vi "Handle Error.vi"(8 "error in (no error)":errorcluster, 11 "Module Data In":refnum<class "Rename.lvclass">) -> (0 "error out":errorcluster, 2 "Stop Module":bool, 3 "Module Data Out":refnum<class "Rename.lvclass">)   [LabVIEW 2015, in "Generic Module Library.lvlib" / "Template G_Module.lvlib" / "Rename.lvclass"]
uses:
  Rename.lvclass
  Template G_Module.lvlib
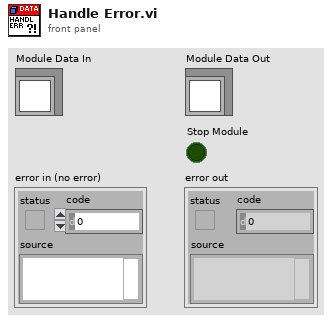
[diagram p1: front panel]
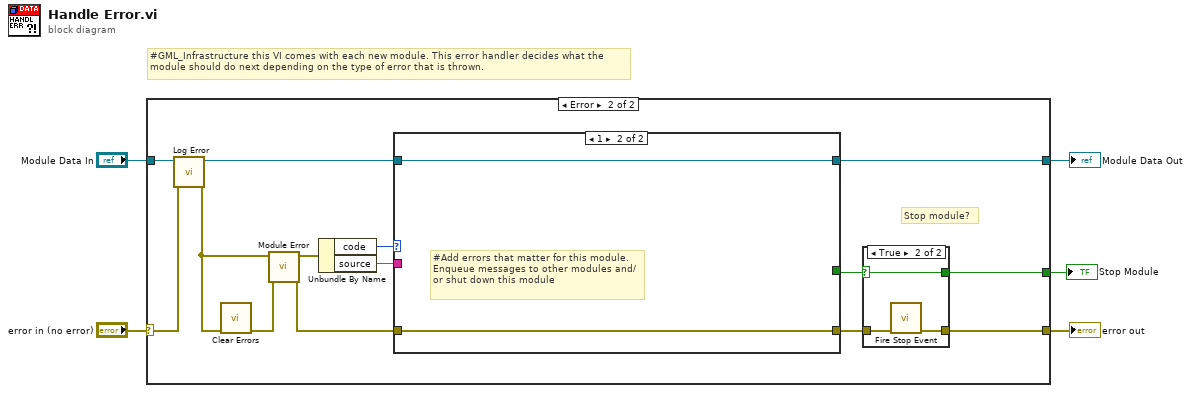
[diagram p0: block diagram]
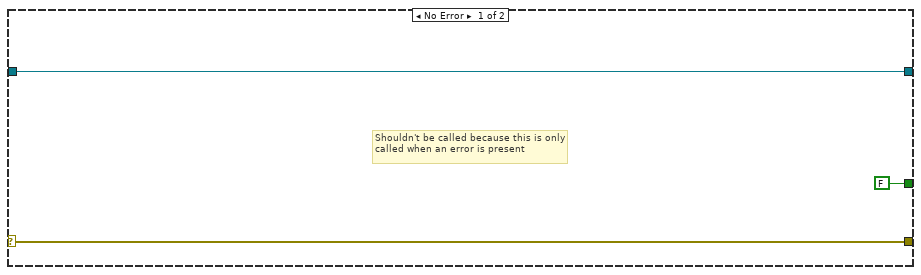
[diagram p2: hidden frame]
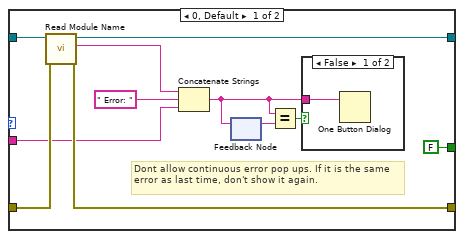
[diagram p4: hidden frame]
diagram:
  # "#GML_Infrastructure this VI comes with each new module. This error handler decides what the module should do next depending on the type of error that is thrown."
  n1 = case shown="Error" "error in (no error)" {
    selector: "error in (no error)" -> [w7 w17]
    tunnel: "Module Data In" -> [w8 w19]
    tunnel: [w7 w15] -> w3
    tunnel: [w8 w22] -> w2
    tunnel: [FALSE w13] -> w1
    frame No Error {
      # "Shouldn't be called because this is only called when an error is present"
    }
    frame Error {
      # "Stop module?"
      n2 = call "Log Error.vi"("error in"=w17, "Module Data In"=w19) -> ("error out"=w10:errorcluster, "Module Data Out"=w18:refnum<class "Rename.lvclass">)  [unwired: 8 in]
      n3 = call <vilib>:"Clear Errors.vi"("error in (no error)"=w10) -> ("error out"=w11:errorcluster)  [unwired: 5 in, 1 out]
      n4 = call "Module Error.vi"("error in"=w11, "Module Error In"=w10) -> ("error out"=w20:errorcluster, "Module Error Out"=w9:errorcluster)  [unwired: 8 in]
      n5 = Unbundle By Name(w9) -> ("code"=w21:i32, "source"=w12:string)
      n6 = case shown="1" w21 {
        tunnel: [w37 w41] -> w22
        tunnel: w18 -> [w38 w41]
        tunnel: w20 -> [w35 w40]
        tunnel: [w34 w40] -> w16
        tunnel: [FALSE _] -> w14
        tunnel: w12 -> [w31 _]
        frame 0, Default {
          # "Dont allow continuous error pop ups. If it is the same error as last time, don't show it again."
          n7 = call-dynamic "Read Module Name.vi"("error in (no error)"=w35, "Rename in"=w38) -> ("error out"=w34:errorcluster, "Module Name"=w32:string, "Rename out"=w37:refnum<class "Rename.lvclass">)  [unwired: 7 in]
          n8 = Concatenate Strings(w32, " Error: " ("string"), w31) -> (w28:string)
          n9 = feedback-in #1(w28) -> ()
          n10 = feedback #1() -> (w29:string)  [unwired: 1 in]
          n11 = Equal?(x=w28, y=w29) -> (x = y?=w30:bool)
          n12 = case shown="False" w30 {
            tunnel: w28 -> [w39 _]
            frame False {
              n13 = One Button Dialog(message=w39) -> ()  [unwired: 1 in, 1 out]
            }
            frame True {
            }
          }
        }
        frame 1 {
          # "#Add errors that matter for this module. Enqueue messages to other modules and/or shut down this module"
        }
      }
      n14 = case shown="True" w14 {
        selector: w14 -> [w24 w25]
        tunnel: [w23 w26] -> w15
        tunnel: w16 -> [w23 w27]
        tunnel: [w24 w25] -> w13
        frame False {
        }
        frame True {
          n15 = call "Fire Stop Event.vi"("error in"=w27) -> ("error out"=w26:errorcluster)  [unwired: 10 in]
        }
      }
    }
  }
  "error out" <- w3
  "Module Data Out" <- w2
  "Stop Module" <- w1
